vi "AlignmentAngle.vi"(10 "Right Distance":dbl, 11 "Left Distance":dbl) -> (2 "Center Distance":dbl, 3 "Angle":dbl)   [LabVIEW 2018]
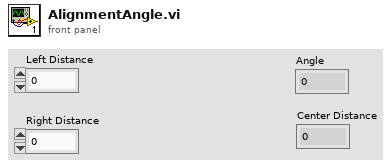
[diagram p1: front panel]
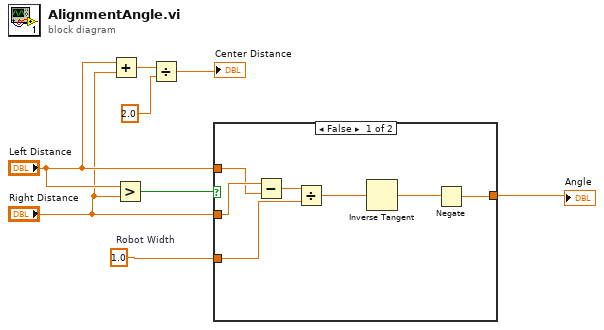
[diagram p0: block diagram]
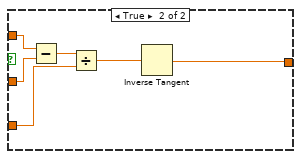
[diagram p2: hidden frame]
diagram:
  w7 = 1.0  # Robot Width
  n1 = Add(x="Left Distance", y="Right Distance") -> (x+y=w3:dbl)
  n2 = Greater?(x="Left Distance", y="Right Distance") -> (0:w8:bool)
  n3 = Divide(x=w3, y=2.0) -> (x/y=→"Center Distance":dbl)
  n4 = case shown="False" w8 {
    tunnel: "Left Distance" -> [w11 w21]
    tunnel: "Right Distance" -> [w12 w20]
    tunnel: w7 -> [w13 w19]
    tunnel: [w9 w16] -> w6
    frame False {
      n5 = Subtract(x=w12, y=w11) -> (x-y=w14:dbl)
      n6 = Divide(x=w14, y=w13) -> (x/y=w15:dbl)
      n7 = Inverse Tangent(1:w15) -> (0:w10:dbl)
      n8 = Negate(x=w10) -> (-x=w9:dbl)
    }
    frame True {
      n9 = Subtract(x=w21, y=w20) -> (x-y=w18:dbl)
      n10 = Divide(x=w18, y=w19) -> (x/y=w17:dbl)
      n11 = Inverse Tangent(1:w17) -> (0:w16:dbl)
    }
  }
  "Angle" <- w6
